vi "6.5.2.vi"() -> ()   [LabVIEW 2018]
panel:
  out "레코드":cluster{"이름":string, "영어성적":dbl, "학번":string}[](array[cluster])
  in  "읽어올 경로":path
  in  "데이터":cluster{"이름":string, "영어성적":dbl, "학번":string}[](array[cluster])
  in  "저장 경로":path
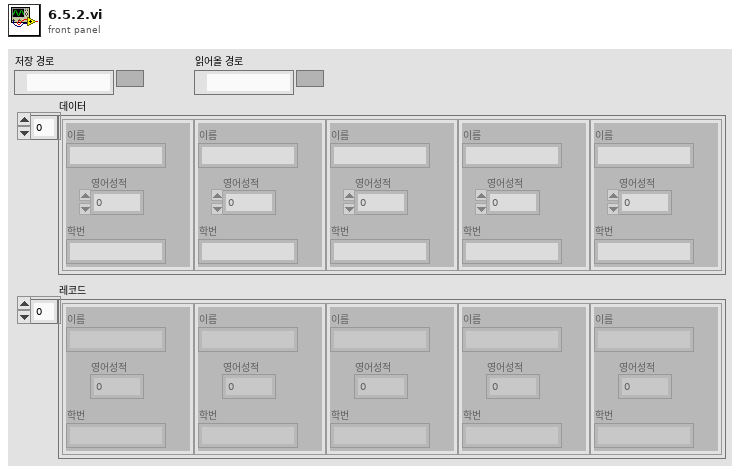
[diagram p1: front panel]
types:
  T1 = enum16{"open", "replace", "create", "open or create", "replace or create", "replace or create with confirmation"}
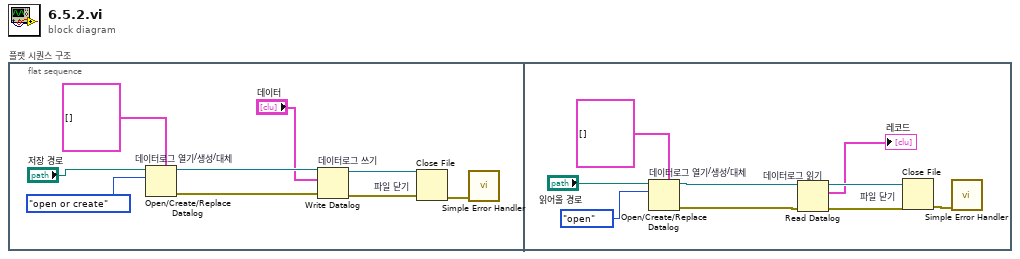
[diagram p0: block diagram]
diagram:
  n1 = flat-sequence "플랫 시퀀스 구조" {
    frame #0 {
      n2 = Open/Create/Replace Datalog "데이터로그 열기/생성/대체"(5:cluster{"이름":string, "영어성적":dbl, "학번":string}[] [] ("데이터 2"), 10:T1."open or create" ("동작(0:open)"), 11:"저장 경로") -> (0:w6:errorcluster, 3:w3:refnum<k1>)  [unwired: 3 in, 1 out]
      n3 = Write Datalog "데이터로그 쓰기"(4:w6, 6:"데이터", 7:w3) -> (0:w5:errorcluster, 3:w1:refnum<k1>)
      n4 = Close File "파일 닫기"(refnum=w1, error in=w5) -> (error out=w7:errorcluster)  [unwired: 1 out]
      n5 = call <vilib>:"Simple Error Handler.vi"("error in (no error)"=w7) -> ()  [unwired: 4 in, 5 out]
    }
    frame #1 {
      n6 = Open/Create/Replace Datalog "데이터로그 열기/생성/대체"(5:cluster{"이름":string, "영어성적":dbl, "학번":string}[] [] ("레코드 2"), 10:T1."open" ("동작(0:open)"), 11:"읽어올 경로") -> (0:w12:errorcluster, 3:w15:refnum<k1>)  [unwired: 3 in, 1 out]
      n7 = Read Datalog "데이터로그 읽기"(4:w12, 7:w15) -> (0:w13:errorcluster, 2:→"레코드":cluster{"이름":string, "영어성적":dbl, "학번":string}[], 3:w14:refnum<k1>)  [unwired: 1 in]
      n8 = Close File "파일 닫기"(refnum=w14, error in=w13) -> (error out=w16:errorcluster)  [unwired: 1 out]
      n9 = call <vilib>:"Simple Error Handler.vi"("error in (no error)"=w16) -> ()  [unwired: 4 in, 5 out]
    }
  }
